vi "Step Response (20 bit).vi"() -> ()   [LabVIEW 2012]
uses:
  Madlib.dll
panel:
  in  "ADC Rate (ms)":T1(ring)
  in  "Step size":dbl=25.0 min=0.0 max=100.0 format="%.2f"
  out "XY Graph 2":cluster{dbl[], "Data Array Out":dbl[]}(graph) caption="Step Response"
  in  "Axis":u32=1 min=1 max=3
  in  "Number of Positions\nto Read":u32=1000 min=1 max=10000
  # "X = 1\nY = 2\nZ = 3"
  # "Percentage of the range of\nmotion to step.  Step will be\ncentered at 50% of the range\nof motion.  A step of 25% will \nmove the axis from 37.5% of\nits range of motion to 62.5%\nof its range of motion."
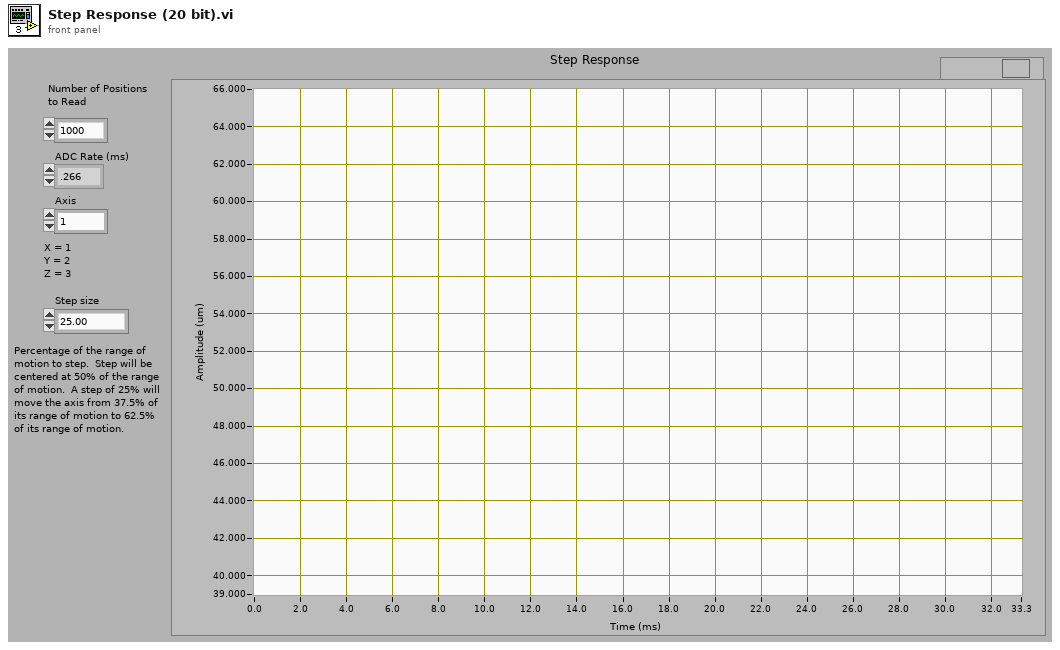
[diagram p1: front panel]
types:
  T1 = enum16{".266", ".5", "1", "2", "10", "16.66", "20"}
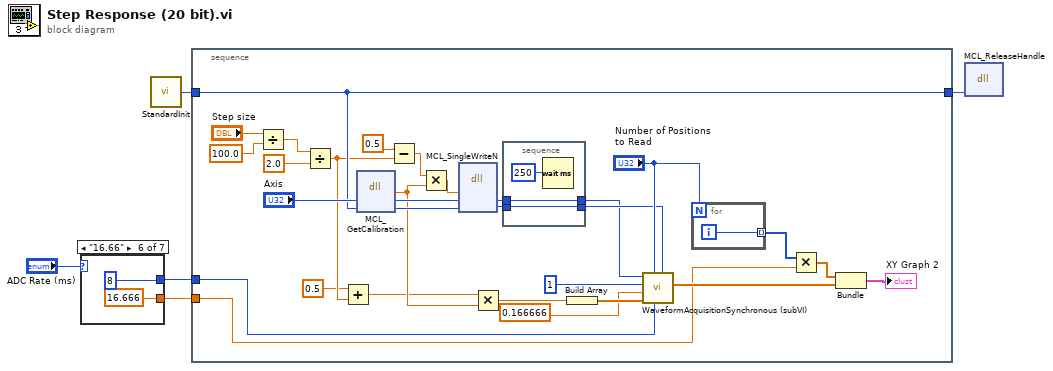
[diagram p0: block diagram]
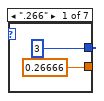
[diagram p2: hidden frame]
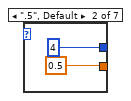
[diagram p3: hidden frame]
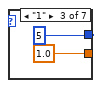
[diagram p4: hidden frame]
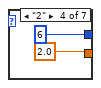
[diagram p5: hidden frame]
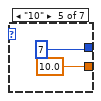
[diagram p6: hidden frame]
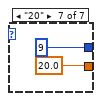
[diagram p7: hidden frame]
diagram:
  n1 = case shown="\"16.66\"" "ADC Rate (ms)" {
    tunnel: [3 4 5 6 7 8 9] -> w2
    tunnel: [0.26666 0.5 1.0 2.0 10.0 16.666 20.0] -> w1
    frame ".266" {
    }
    frame ".5", Default {
    }
    frame "1" {
    }
    frame "2" {
    }
    frame "10" {
    }
    frame "16.66" {
    }
    frame "20" {
    }
  }
  n2 = call "StandardInit.vi"() -> ("Outgoing Handle"=w5:i32)  [unwired: 1 in]
  n3 = stacked-sequence {
    tunnel: w5 -> [w32]
    tunnel: [w32] -> w4
    tunnel: w2 -> [w21]
    tunnel: w1 -> [w20]
    frame #0 {
      n4 = Divide(x="Step size", y=100.0) -> (x/y=w23:dbl)
      n5 = Divide(x=w23, y=2.0) -> (x/y=w28:dbl)
      n6 = Add(x=0.5, y=w28) -> (x+y=w26:dbl)
      n7 = dll-call lib="C:/Users/Labview/Desktop/SRR/Madlib_x64/Labview Examples/MADLib.dll" fn="MCL_GetCalibration"("axis"="Axis", "handle"=w32) -> (w34:dbl, "axis"=w38:u32, "handle"=w39:i32)  [unwired: 3 in, 2 out]
      n8 = Subtract(x=0.5, y=w28) -> (x-y=w31:dbl)
      n9 = Multiply(x=w31, y=w34) -> (x*y=w33:dbl)
      n10 = dll-call lib="C:/Users/Labview/Desktop/SRR/Madlib_x64/Labview Examples/MADLib.dll" fn="MCL_SingleWriteN"("position"=w33, "axis"=w38, "handle"=w39) -> ("axis"=w37:u32, "handle"=w41:i32)  [unwired: 5 in, 2 out]
      n11 = Multiply(x=w26, y=w34) -> (x*y=w42:dbl)
      n12 = stacked-sequence {
        tunnel: [w51] -> w36
        tunnel: w41 -> [w51]
        tunnel: [w50] -> w35
        tunnel: w37 -> [w50]
        frame #0 {
          n13 = Wait (ms)(milliseconds to wait=250) -> ()  [unwired: 1 out]
        }
      }
      n14 = Build Array(w42) -> (w46:dbl[])
      n15 = call "WaveformAcquisitionSynchronous (subVI).vi"("Handle"=w36, "ADC Rate (ms)"=w21, "Number of Positions to Read"="Number of Positions\nto Read", "Data Array In"=w46, "DAC Rate (ms)"=0.166666, "Number of Steps"=1, "Axis"=w35) -> ("Data Array Out"=w43:dbl[])  [unwired: 2 in, 1 out]
      n16 = for {
        N: "Number of Positions\nto Read" -> [_]
        tunnel: [w53] -> w49 mode=indexing
        i -> [w53]
      }
      n17 = Multiply(x=w49, y=w20) -> (x*y=w48:dbl[])
      n18 = Bundle(w48, "Data Array Out"=w43) -> (→"XY Graph 2":cluster{dbl[], "Data Array Out":dbl[]})  [unwired: 1 in]
    }
  }
  n19 = dll-call lib="C:/Users/Labview/Desktop/SRR/Madlib_x64/Labview Examples/MADLib.dll" fn="MCL_ReleaseHandle"("handle"=w4) -> ()  [unwired: 5 in, 2 out]
